vi "Parameter generator.vi"(8 "Mode":T1, 9 "Step/Iterations":dbl, 10 "To":dbl, 11 "From":dbl) -> (0 "error out":errorcluster, 2 "Size of the array":i32, 3 "Array of parameter values":string[](array[string]))   [LabVIEW 2020, in "TALOS.lvlib" / "Run Utilities.lvlib" / "Scan SBlock.lvclass"]
uses:
  Scan SBlock.lvclass
  Advanced Panel Parameter Mode.ctl
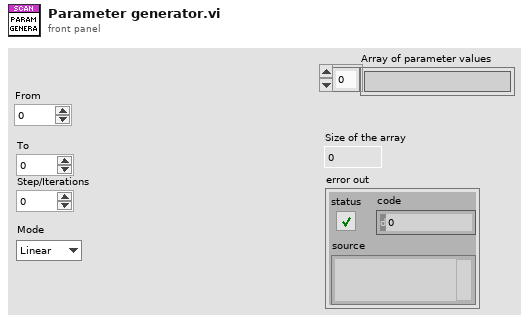
[diagram p1: front panel]
types:
  T1 = typedef "TALOS.lvlib/Run Utilities.lvlib/Scan SBlock.lvclass/Advanced Panel Parameter Mode.ctl" = enum16{"Linear", "Log", "LINKED"}
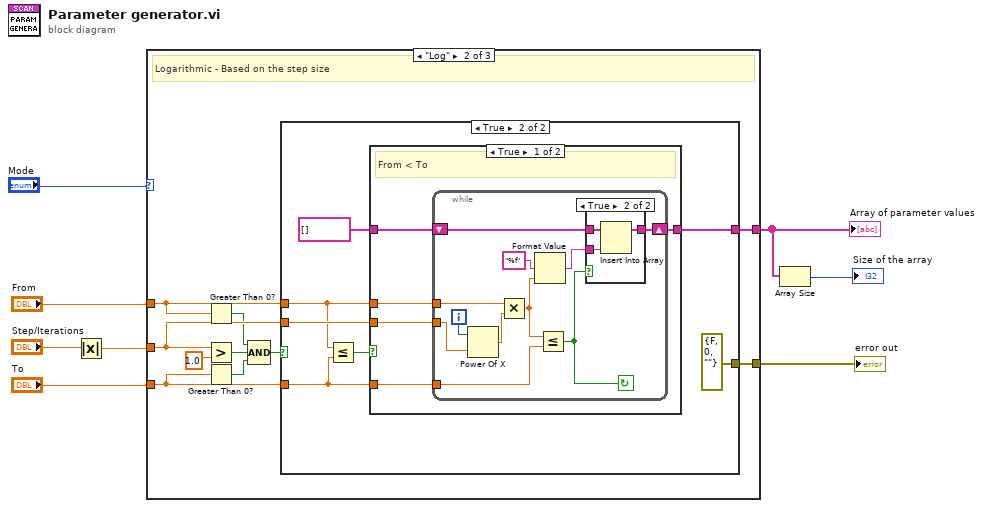
[diagram p0: block diagram]
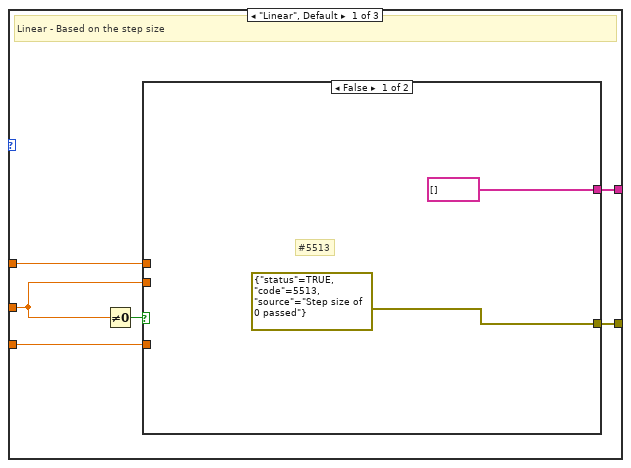
[diagram p2: hidden frame]
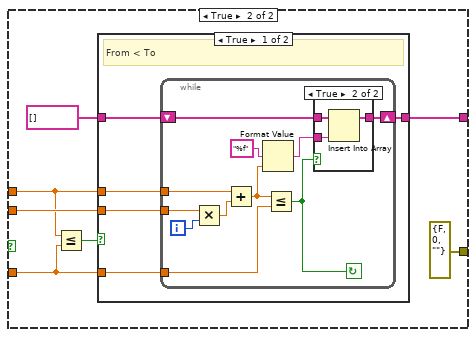
[diagram p3: hidden frame]
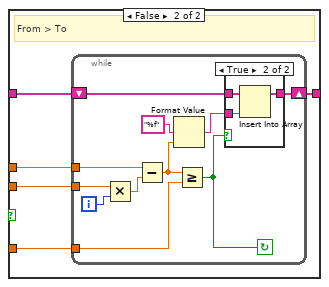
[diagram p5: hidden frame]
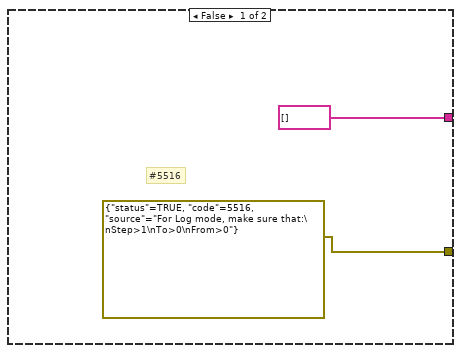
[diagram p7: hidden frame]
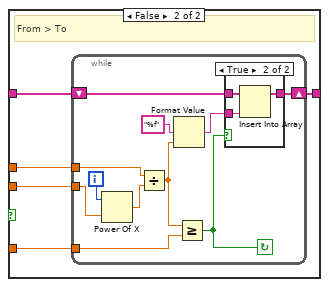
[diagram p9: hidden frame]
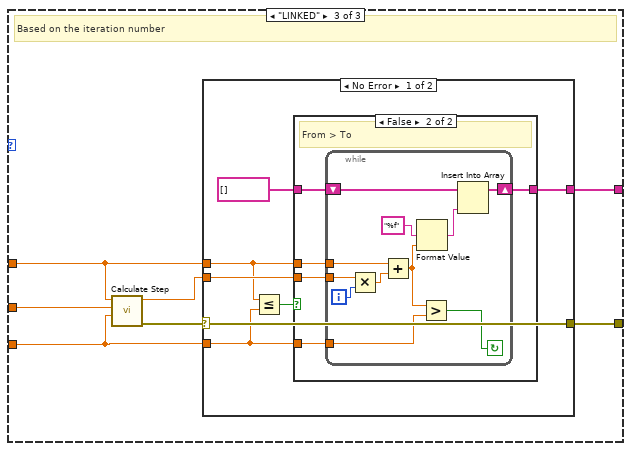
[diagram p11: hidden frame]
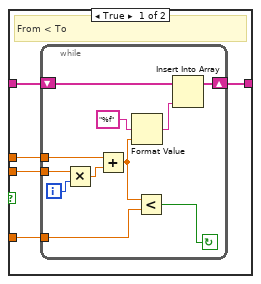
[diagram p12: hidden frame]
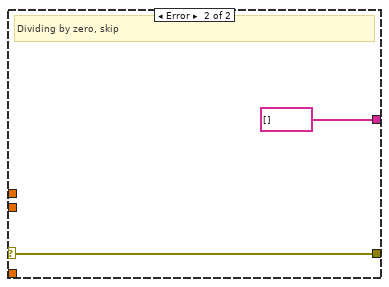
[diagram p13: hidden frame]
diagram:
  n1 = Absolute Value(x="Step/Iterations") -> (abs(x)=w2:dbl)
  n2 = case shown="\"Log\"" "Mode" {
    tunnel: "To" -> [w12 w69 w123]
    tunnel: w2 -> [w10 w71 w124]
    tunnel: "From" -> [w13 w68 w127]
    tunnel: [w14 w73 w126] -> w8
    tunnel: [w11 w72 w125] -> w6
    frame "Linear", Default {
      # "Linear - Based on the step size"
      n3 = Not Equal To 0?(x=w10) -> (x != 0?=w9:bool)
      n4 = case shown="False" w9 {
        tunnel: [string[] [] w22] -> w14
        tunnel: w13 -> [_ w18]
        tunnel: w12 -> [_ w17]
        tunnel: [errorcluster {"status"=TRUE, "code"=5513, "source"="Step size of 0 passed"} ("error out") errorcluster {"status"=FALSE, "code"=0, "source"=""} ("error IO")] -> w11
        tunnel: w10 -> [_ w20]
        frame False {
          # "#5513"
        }
        frame True {
          n5 = Less Or Equal?(x=w18, y=w17) -> (x <= y?=w19:bool)
          n6 = case shown="True" w19 {
            tunnel: string[] [] -> [w28 w48]
            tunnel: [w27 w47] -> w22
            tunnel: w18 -> [w26 w46]
            tunnel: w17 -> [w25 w45]
            tunnel: w20 -> [w24 w44]
            frame True {
              # "From < To"
              n7 = while {
                tunnel: w26 -> [w37]
                tunnel: w24 -> [w34]
                tunnel: w25 -> [w33]
                shift-right: [w35] -> w27
                shift-left: w28 -> [w36]
                i -> [w39]
                stop <- w29 continue-if-true
                n8 = Multiply(x=w34, y=w39) -> (x*y=w38:dbl)
                n9 = Add(x=w37, y=w38) -> (x+y=w31:dbl)
                n10 = Format Value(format string="%f", value (0)=w31) -> (output string=w30:string)  [unwired: 1 in]
                n11 = Less Or Equal?(x=w31, y=w33) -> (x <= y?=w29:bool)
                n12 = case shown="True" w29 {
                  tunnel: w36 -> [w40 w43]
                  tunnel: [w40 w42] -> w35
                  tunnel: w30 -> [_ w41]
                  frame False {
                  }
                  frame True {
                    n13 = Insert Into Array(array=w43, new element=w41) -> (w42:string[])  [unwired: 1 in]
                  }
                }
              }
            }
            frame False {
              # "From > To"
              n14 = while {
                tunnel: w46 -> [w57]
                tunnel: w44 -> [w54]
                tunnel: w45 -> [w53]
                shift-right: [w55] -> w47
                shift-left: w48 -> [w56]
                i -> [w59]
                stop <- w49 continue-if-true
                n15 = Multiply(x=w54, y=w59) -> (x*y=w58:dbl)
                n16 = Subtract(x=w57, y=w58) -> (x-y=w51:dbl)
                n17 = Format Value(format string="%f", value (0)=w51) -> (output string=w50:string)  [unwired: 1 in]
                n18 = Greater Or Equal?(x=w51, y=w53) -> (x >= y?=w49:bool)
                n19 = case shown="True" w49 {
                  tunnel: w56 -> [w60 w63]
                  tunnel: [w60 w62] -> w55
                  tunnel: w50 -> [_ w61]
                  frame False {
                  }
                  frame True {
                    n20 = Insert Into Array(array=w63, new element=w61) -> (w62:string[])  [unwired: 1 in]
                  }
                }
              }
            }
          }
        }
      }
    }
    frame "Log" {
      # "Logarithmic - Based on the step size"
      n21 = Greater Than 0?(x=w68) -> (x > 0?=w67:bool)
      n22 = Greater?(x=w71, y=1.0) -> (0:w66:bool)
      n23 = Greater Than 0?(x=w69) -> (x > 0?=w65:bool)
      n24 = Compound Arithmetic op=AND(w67, w66, w65) -> (w64:bool)
      n25 = case shown="True" w64 {
        tunnel: [string[] [] w81] -> w73
        tunnel: w68 -> [_ w77]
        tunnel: w69 -> [_ w76]
        tunnel: [errorcluster {"status"=TRUE, "code"=5516, "source"="For Log mode, make sure that:\nStep>1\nTo>0\nFrom>0"} ("error out") errorcluster {"status"=FALSE, "code"=0, "source"=""} ("error IO")] -> w72
        tunnel: w71 -> [_ w79]
        frame False {
          # "#5516"
        }
        frame True {
          n26 = Less Or Equal?(x=w77, y=w76) -> (x <= y?=w78:bool)
          n27 = case shown="True" w78 {
            tunnel: string[] [] -> [w87 w107]
            tunnel: [w86 w106] -> w81
            tunnel: w77 -> [w83 w103]
            tunnel: w76 -> [w85 w105]
            tunnel: w79 -> [w84 w104]
            frame True {
              # "From < To"
              n28 = while {
                tunnel: w84 -> [w91]
                tunnel: w85 -> [w96]
                shift-right: [w97] -> w86
                shift-left: w87 -> [w98]
                tunnel: w83 -> [w89]
                i -> [w88]
                stop <- w93 continue-if-true
                n29 = Power Of X(1:w91, 2:w88) -> (0:w92:dbl)
                n30 = Multiply(x=w89, y=w92) -> (x*y=w90:dbl)
                n31 = Format Value(format string="%f", value (0)=w90) -> (output string=w94:string)  [unwired: 1 in]
                n32 = Less Or Equal?(x=w90, y=w96) -> (x <= y?=w93:bool)
                n33 = case shown="True" w93 {
                  tunnel: w98 -> [w99 w102]
                  tunnel: [w99 w101] -> w97
                  tunnel: w94 -> [_ w100]
                  frame False {
                  }
                  frame True {
                    n34 = Insert Into Array(array=w102, new element=w100) -> (w101:string[])  [unwired: 1 in]
                  }
                }
              }
            }
            frame False {
              # "From > To"
              n35 = while {
                tunnel: w104 -> [w109]
                tunnel: w105 -> [w116]
                shift-right: [w117] -> w106
                shift-left: w107 -> [w118]
                tunnel: w103 -> [w111]
                i -> [w108]
                stop <- w113 continue-if-true
                n36 = Power Of X(1:w109, 2:w108) -> (0:w112:dbl)
                n37 = Divide(x=w111, y=w112) -> (x/y=w110:dbl)
                n38 = Format Value(format string="%f", value (0)=w110) -> (output string=w114:string)  [unwired: 1 in]
                n39 = Greater Or Equal?(x=w110, y=w116) -> (x >= y?=w113:bool)
                n40 = case shown="True" w113 {
                  tunnel: w118 -> [w119 w122]
                  tunnel: [w119 w121] -> w117
                  tunnel: w114 -> [_ w120]
                  frame False {
                  }
                  frame True {
                    n41 = Insert Into Array(array=w122, new element=w120) -> (w121:string[])  [unwired: 1 in]
                  }
                }
              }
            }
          }
        }
      }
    }
    frame "LINKED" {
      # "Based on the iteration number"
      n42 = call "Calculate Step.vi"("To"=w123, "No of iterations"=w124, "From"=w127) -> ("error out"=w129:errorcluster, "Step"=w128:dbl)  [unwired: 7 in]
      n43 = case shown="No Error" w129 {
        selector: w129 -> [w133 w169]
        tunnel: w128 -> [w135 _]
        tunnel: w127 -> [w131 _]
        tunnel: [w134 string[] []] -> w126
        tunnel: [w133 w169] -> w125
        tunnel: w123 -> [w132 _]
        frame No Error {
          n44 = Less Or Equal?(x=w131, y=w132) -> (x <= y?=w130:bool)
          n45 = case shown="False" w130 {
            tunnel: string[] [] -> [w141 w157]
            tunnel: w135 -> [w140 w156]
            tunnel: w131 -> [w139 w155]
            tunnel: [w138 w154] -> w134
            tunnel: w132 -> [w137 w153]
            frame True {
              # "From < To"
              n46 = while {
                tunnel: w139 -> [w150]
                tunnel: w140 -> [w147]
                shift-right: [w148] -> w138
                shift-left: w141 -> [w149]
                tunnel: w137 -> [w146]
                i -> [w152]
                stop <- w145 continue-if-true
                n47 = Multiply(x=w147, y=w152) -> (x*y=w151:dbl)
                n48 = Add(x=w150, y=w151) -> (x+y=w143:dbl)
                n49 = Format Value(format string="%f", value (0)=w143) -> (output string=w142:string)  [unwired: 1 in]
                n50 = Less?(x=w143, y=w146) -> (x < y?=w145:bool)
                n51 = Insert Into Array(array=w149, new element=w142) -> (w148:string[])  [unwired: 1 in]
              }
            }
            frame False {
              # "From > To"
              n52 = while {
                tunnel: w155 -> [w166]
                tunnel: w156 -> [w163]
                shift-right: [w164] -> w154
                shift-left: w157 -> [w165]
                tunnel: w153 -> [w162]
                i -> [w168]
                stop <- w161 continue-if-true
                n53 = Multiply(x=w163, y=w168) -> (x*y=w167:dbl)
                n54 = Add(x=w166, y=w167) -> (x+y=w159:dbl)
                n55 = Format Value(format string="%f", value (0)=w159) -> (output string=w158:string)  [unwired: 1 in]
                n56 = Greater?(x=w159, y=w162) -> (0:w161:bool)
                n57 = Insert Into Array(array=w165, new element=w158) -> (w164:string[])  [unwired: 1 in]
              }
            }
          }
        }
        frame Error {
          # "Dividing by zero, skip"
        }
      }
    }
  }
  "error out" <- w6
  "Array of parameter values" <- w8
  n58 = Array Size(array=w8) -> (size(s)=→"Size of the array":i32)
